vi "Logger.TestLauncher.vi"() -> ()   [LabVIEW 2016, in "Logger.DSC.lvclass"]
uses:
  Logger.DSC.lvclass
  <vilib>/JKI/JKI SMO/SMO/Typedefs/SMOState --Enum.ctl
  C:/Program Files (x86)/National Instruments/LabVIEW 2016/vi.lib/JKI/JKI SMO/SMO/SMO.lvclass
  <vilib>/JKI/JKI SMO/SMO/SMO.lvclass
panel:
  out "Data":variant
  out "x+1":i32
  out "time":u32
  out "read":u32
  out "write":u32
  in  "shared variable refnum in":refnum<k21>
  in  "Write":bool
  in  "test value":dbl
  out "SMO State":T1
  out "error out":errorcluster
  in  "Stop":bool
  # "Logger Test Launcher (DSC)"
  # "For instructions on how to use the JKI State Machine Objects, examples and video tutorials, visit:\nhttp://jki.net/state-machine-objects/\n\nJKI State Machine Objects™\nhttp://jki.net/state-machine-objects/\nCopyright (C) 2005-2015, JKI <info@jki.net>\nALL RIGHTS RESERVED"
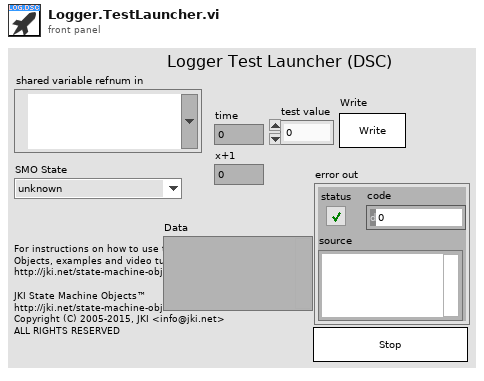
[diagram p1: front panel]
types:
  T1 = typedef "SMO.lvclass/SMOState --Enum.ctl" = enum16{"unknown", "Created", "Started", "Stopped"}
  T2 = typedef "SMO.lvclass/Public Events.ctl" = cluster{"Error":refnum<user-event>, "State":refnum<user-event>, "Reserve State":refnum<user-event>}
  T3 = typedef "Logger.DSC.lvclass/PublicEvents--Cluster.ctl" = cluster{"Read Variable":refnum<user-event>}
  T4 = cluster{"Event Registration Refnum":refnum<event-registration>}
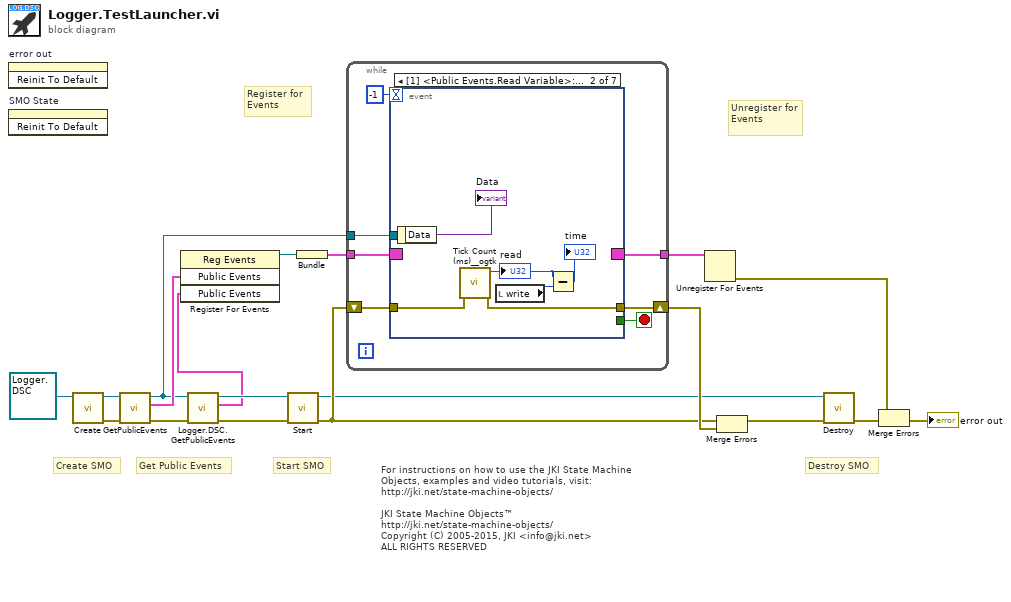
[diagram p0: block diagram]
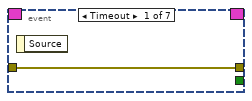
[diagram p2: hidden frame]
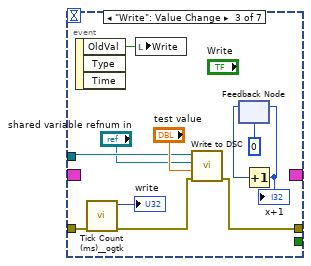
[diagram p3: hidden frame]
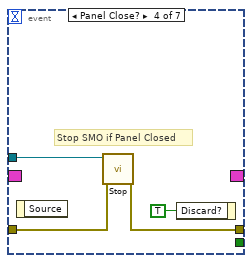
[diagram p4: hidden frame]
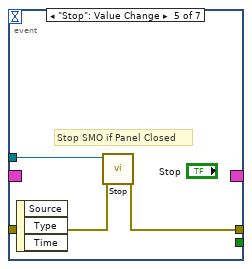
[diagram p5: hidden frame]
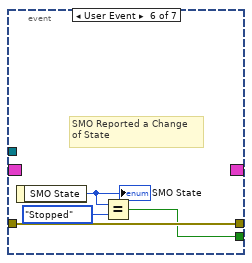
[diagram p6: hidden frame]
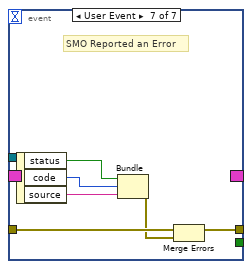
[diagram p7: hidden frame]
diagram:
  # "For instructions on how to use the JKI State Machine Objects, examples and video tutorials, visit:\nhttp://jki.net/state-machine-objects/\n\nJKI State Machine Objects™\nhttp://jki.net/state-machine-objects/\nCopyright (C) 2005-2015, JKI <info@jki.net>\nALL RIGHTS RESERVED"
  # "Get Public Events"
  # "Start SMO"
  # "Destroy SMO"
  # "Create SMO"
  # "Unregister for Events"
  # "Register for Events"
  n1 = invoke on="error out" class="Clust (strict)" method="Reinit To Default"() -> ()  [unwired: 3 in, 3 out]
  n2 = invoke on="SMO State" class="Enum (strict)" method="Reinit To Default"() -> ()  [unwired: 3 in, 3 out]
  n3 = call <vilib>:"Create.vi"("SMO"=refnum<class "Logger.DSC.lvclass"> refnum ("SMO.Template.lvclass")) -> ("error out"=w8:errorcluster, "SMO out"=w9:refnum<class "Logger.DSC.lvclass">)  [unwired: 8 in, 1 out]
  n4 = call <vilib>:"GetPublicEvents.vi"("error in (no error)"=w8, "SMO"=w9) -> ("error out"=w4:errorcluster, "Public Events"=w7:T2, "SMO out"=w5:refnum<class "Logger.DSC.lvclass">)  [unwired: 7 in]
  n5 = call "Logger.DSC.GetPublicEvents.vi"("error in (no error)"=w4, "Logger"=w5) -> ("error out"=w3:errorcluster, "Public Events"=w1:T3, "Logger out"=w2:refnum<class "Logger.DSC.lvclass">)  [unwired: 7 in]
  n6 = register-events(w7, w1) -> (reference out=w6:refnum<event-registration>)  [unwired: 2 in, 1 out]
  n7 = call <vilib>:"Start.vi"("error in (no error)"=w3, "SMO"=w2) -> ("error out"=w12:errorcluster, "SMO out"=w10:refnum<class "Logger.DSC.lvclass">)  [unwired: 8 in]
  n8 = Bundle("Event Registration Refnum"=w6) -> (w18:T4)  [unwired: 1 in]
  n9 = while {
    shift-right: [w25] -> w17
    shift-left: w12 -> [w24]
    tunnel: w18 -> [w23]
    tunnel: [w22] -> w19
    tunnel: w5 -> [w21]
    stop <- w26 stop-if-true
    n10 = event shown="[1] <Public Events.Read Variable>: User Event" {
      selector: w23 -> [_ _ _ _ _ _ _]
      dyn-events: [_ _ _ _ _ _ _] -> w22
      timeout: -1 -> [_ _ _ _ _ _ _]
      tunnel: [_ _ _ _ _ w52 _] -> w26
      tunnel: w21 -> [_ _ w35 w48 w51 _ _]
      tunnel: [w27 w32 w36 w47 w50 w55 w59] -> w25
      tunnel: w24 -> [w27 w33 w44 w46 w49 w55 w57]
      event Timeout {
        n11 = event-data() -> ()  [unwired: 1 in, 1 out]
      }
      event User Event {
        n12 = event-data() -> ("Data"=→"Data":variant)  [unwired: 1 in]
        n13 = call <userlib>:"Tick Count (ms)__ogtk.vi"("error in (no error)"=w33) -> ("error out"=w32:errorcluster, "millisecond timer value"=w30:u32)  [unwired: 9 in]
        "read" <- w30
        n14 = local read "write"() -> (w31:u32)
        n15 = Subtract(x=w30, y=w31) -> (x-y=→"time":u32)
      }
      event "Write": Value Change {
        n16 = event-data() -> ("OldVal"=w39:bool)  [unwired: 1 in, 2 out]
        n17 = call <userlib>:"Tick Count (ms)__ogtk.vi"("error in (no error)"=w44) -> ("error out"=w37:errorcluster, "millisecond timer value"=→"write":u32)  [unwired: 9 in]
        n18 = local write "Write"(w39) -> ()
        n19 = call-dynamic "Write to DSC.vi"("error in (no error)"=w37, "Variant"="test value", "Process name"="shared variable refnum in", "Logger in"=w35) -> ("error out"=w36:errorcluster)  [unwired: 6 in, 1 out]
        n20 = feedback #1(0) -> (w41:i32)
        n21 = Increment(x=w41) -> (x+1=w42:i32)
        "x+1" <- w42
        n22 = feedback-in #1(w42) -> ()
      }
      event Panel Close? {
        # "Stop SMO if Panel Closed"
        n23 = event-data() -> ()  [unwired: 1 in, 1 out]
        n24 = call <vilib>:"Stop.vi"("error in (no error)"=w46, "SMO"=w48) -> ("error out"=w47:errorcluster)  [unwired: 8 in, 1 out]
        n25 = event-data("Discard?"=TRUE ("OK")) -> ()  [unwired: 1 in, 1 out]
      }
      event "Stop": Value Change {
        # "Stop SMO if Panel Closed"
        n26 = event-data() -> ()  [unwired: 1 in, 3 out]
        n27 = call <vilib>:"Stop.vi"("error in (no error)"=w49, "SMO"=w51) -> ("error out"=w50:errorcluster)  [unwired: 8 in, 1 out]
      }
      event User Event {
        # "SMO Reported a Change\nof State"
        n28 = event-data() -> ("SMO State"=w54:T1)  [unwired: 1 in]
        "SMO State" <- w54
        n29 = Equal?(x=w54, y=SMOState_--Enum."Stopped") -> (x = y?=w52:bool)
      }
      event User Event {
        # "SMO Reported an Error"
        n30 = event-data() -> ("status"=w58:bool, "code"=w61:i32, "source"=w60:string)  [unwired: 1 in]
        n31 = Bundle("status"=w58, "code"=w61, "source"=w60) -> (w56:errorcluster)  [unwired: 1 in]
        n32 = Merge Errors(w57, w56) -> (w59:errorcluster)
      }
    }
  }
  n33 = Unregister For Events(event registration refnum=w19) -> (error out=w16:errorcluster)  [unwired: 1 in]
  n34 = Merge Errors(w12, w17) -> (w11:errorcluster)
  n35 = call <vilib>:"Destroy.vi"("error in (no error)"=w11, "SMO"=w10) -> ("error out"=w14:errorcluster)  [unwired: 9 in]
  n36 = Merge Errors(w16, w14) -> (→"error out":errorcluster)
